vi "ImagerForFlowbit4.vi"() -> ()   [LabVIEW 2011]
uses:
  <vilib>/Platform/TimedLoop/XDataNode/timing_clust.ctl
  <vilib>/Platform/TimedLoop/XDataNode/nitl_modes.ctl
  <vilib>/Platform/TimedLoop/XDataNode/wakeup.ctl
  <vilib>/Analysis/1siggen.llb/Riffle Array (I32).vi
  <vilib>/Platform/TimedLoop/XDataNode/XDataNode.xnode
  <vilib>/Analysis/NI_AALBase.lvlib
  <vilib>/vision/NI_Vision_Development_Module.lvlib
  <vilib>/Platform/TimedLoop/XDataNode/XDNodeRunTimeDep.lvlib
panel:
  out "停止循环":bool
  in  "Stimuli":i64=5
  in  "选项卡控件":enum32{"前面板", "参数设置", "OnLineMap"}(tab)
  out "log":string
  out "Stim_ID":i32(listbox)=1
  in  "开始/暂停":bool=TRUE
  in  "停止":bool
  out "重排的 Stim ID":i32[](array[numeric]) caption="重排的{X}"
  out "block":i32
  out "队列中元素数量":i32
  out "Image 2":T1(plugin-control)
  in  "热图":bool
  out "循环持续时间":i64
  out "Recording":bool
  out "grabLoop":i32
  in  "address":i16=888 caption="地址" format="%.0x"
  in  "SaveParameter":bool
  in  "Pra_binType":enum16{"Extract", "Resample"}(ring)
  in  "Pra_FramesPerStim":i64=16
  in  "Pra_Blk目录":path=path "D:/Expt/test"
  in  "Pra_文件名":string="G4_E02"
  in  "Pra_TimeForPrepare(ms)":u32=1000
  in  "Pra_stim ID":u8[](array[numeric])=[0, 2, 4, 6, 8]
  in  "Pra_blk总数":i32=500
  in  "Pra_stim protocol":T2(array[ring])=[enum."prep stim", enum."wait respirator", enum."show stim", enum."recording data", enum."Blank stim", enum."ISI"]
  in  "Pra_blank stim":u8
  in  "Pra_wait（ms）":u32=10
  in  "Pra_ISI（ms）":u32=8000
  in  "Pra_FrameBin":i32=25
  in  "Pra_datatype":u16(ring)=13 items=["U8"=11, "I16"=12, "U32"=13, "SGL"=14]
  in  "FrameWidth":i64=704
  in  "FrameHeight":i64=576
  in  "LoadParameter":bool
  in  "Pra_bin":enum16{"1*1", "2*2"}(ring)
  in  "Pra_DR/R parameter":T3={"frame_zero_0"=0, "frame_zero_1"=1, "frame_0"=3, "frame_1"=15}
  in  "Pra_OnlineMap":cluster{"数组 1":i32[], "数组 2":i32[]}[](array[cluster])=[{"数组 1"=[2], "数组 2"=[6]}, {"数组 1"=[4], "数组 2"=[8]}, {"数组 1"=[2, 6], "数组 2"=[4, 8]}, {"数组 1"=[2, 4, 6, 8], "数组 2"=[0]}, {"数组 1"=[2, 4], "数组 2"=[6, 8]}]
  # "-"
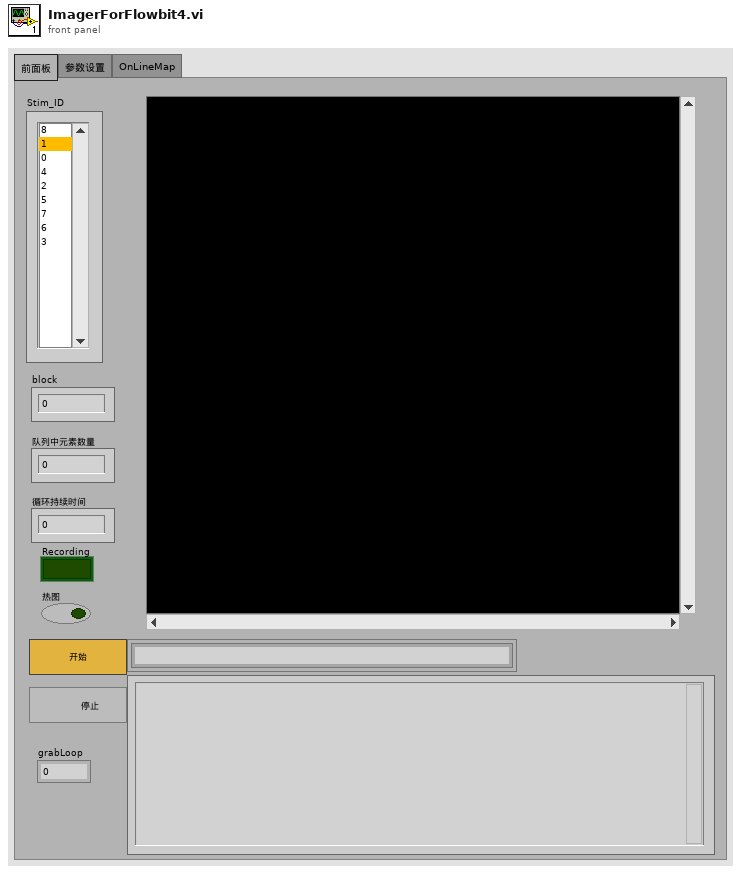
[diagram p1: front panel]
types:
  T1 = typedef "IMAQ Image.ctl" = refnum<image>
  T2 = enum16{"wait", "prep stim", "show stim", "wait respirator", "recording data", "Blank stim", "wait heart", "ISI", "DR/R", "wait calibrate", "openLightShutter", "closeLightShutter"}[]
  T3 = cluster{"frame_zero_0":i32, "frame_zero_1":i32, "frame_0":i32, "frame_1":i32}
  T4 = typedef "Image Type" = u32
  T5 = enum16{"Disable External Trigger", "Enable External Trigger"}
  T6 = enum32{"Auto Detect", "RoadRunner", "Raven", "R64"}
  T7 = typedef "XDNodeRunTimeDep.lvlib/timing_clust.ctl" = cluster{"Expected End [f-1]":u64, "Actual End [f-1]":u64, "Finished Late? [f-1]":bool, "Expected End [i-1]":u64, "Actual End [i-1]":u64, "Finished Late? [i-1]":bool, "Expected Start [i]":u64, "Actual Start [i]":u64, "Expected Start [f]":u64, "Actual Start [f]":u64, "Source Name":string, "Structure Name":string, "Period":i64, "Deadline":i64, "Offset":i64, "Start":i64, "Priority":i32, "Timeout":i32, "Mode":T8, "Wakeup Reason":T9, "Error":errorcluster, "Source Type":string, "Secondary Source Type":string, "Global End Time":u64, "Global Start Time":u64, "Frame Duration":u64, "Iteration Duration":u64, "Assigned CPU":i32, "I/O Scan Engine Mode":u32}
  T8 = typedef "XDNodeRunTimeDep.lvlib/nitl_modes.ctl" = enum32{"No Change", "Process missed periods, maintain original phase", "Discard missed periods, maintain original phase", "Process missed periods, ignore original phase", "Discard missed periods, ignore original phase"}
  T9 = typedef "XDNodeRunTimeDep.lvlib/wakeup.ctl" = enum32{"Normal", "Aborted", "Asynchronous wakeup", "Timing source error", "Timed loop error", "Timeout"}
  T10 = enum8{"Enabled", "Disabled", "Disabled and Grayed Out"}
  T11 = enum16{"open", "replace", "create", "open or create", "replace or create", "replace or create with confirmation"}
  T12 = enum16{"big-endian, network order", "native, host order", "little-endian"}
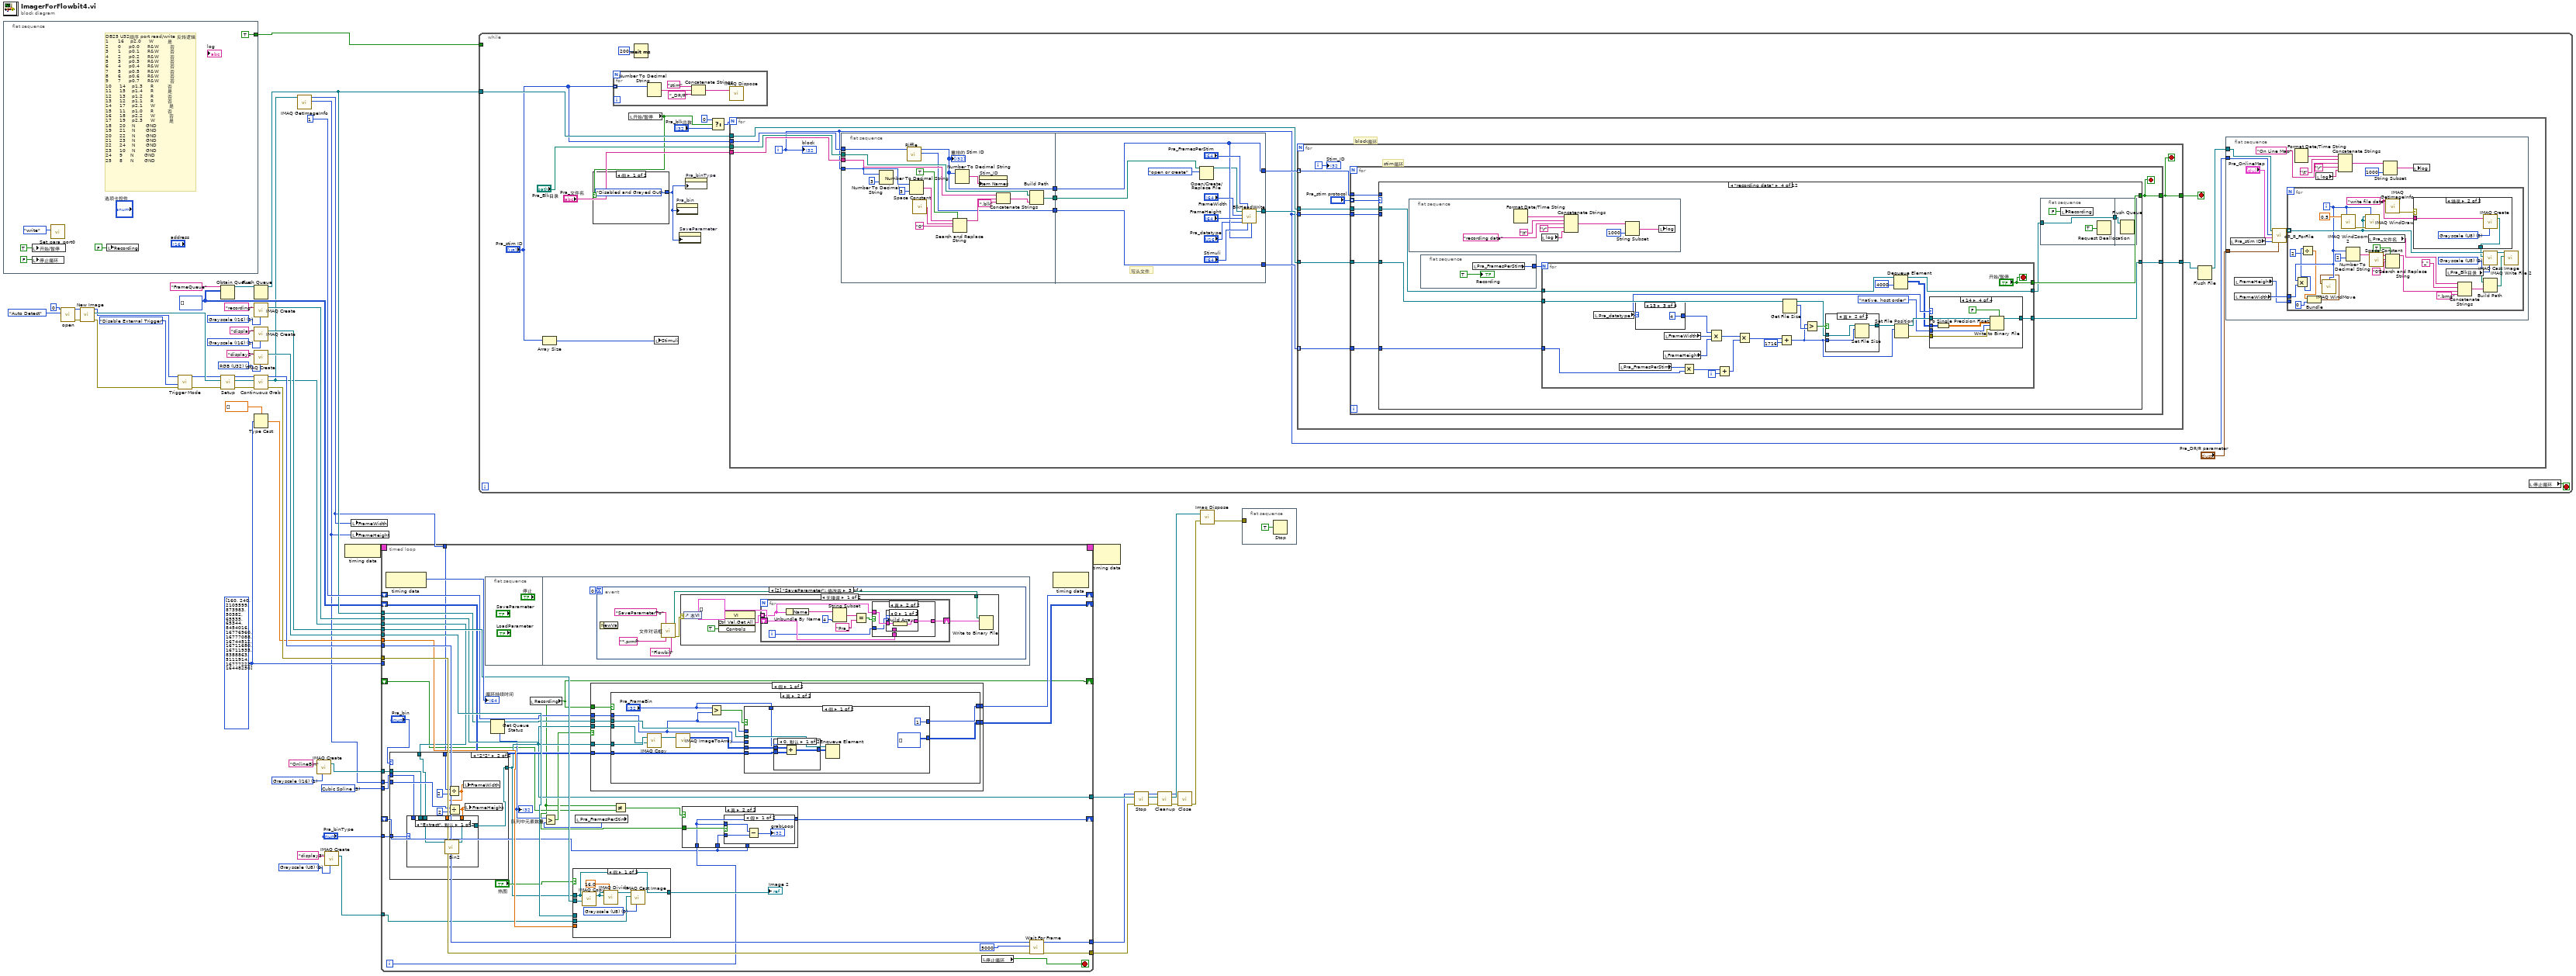
[diagram p0: block diagram]
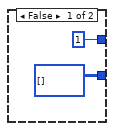
[diagram p4: hidden frame]
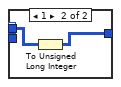
[diagram p5: hidden frame]
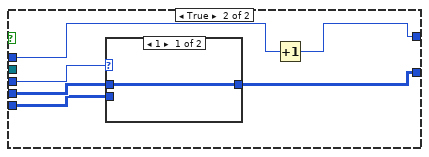
[diagram p6: hidden frame]
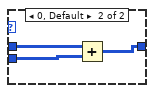
[diagram p7: hidden frame]
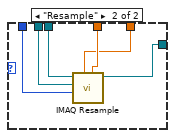
[diagram p10: hidden frame]
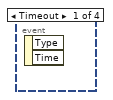
[diagram p11: hidden frame]
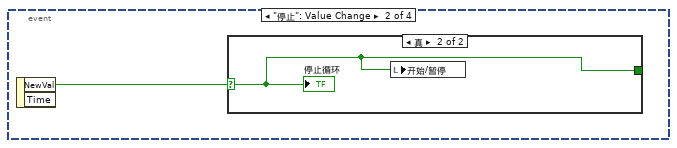
[diagram p12: hidden frame]
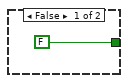
[diagram p13: hidden frame]
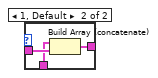
[diagram p15: hidden frame]
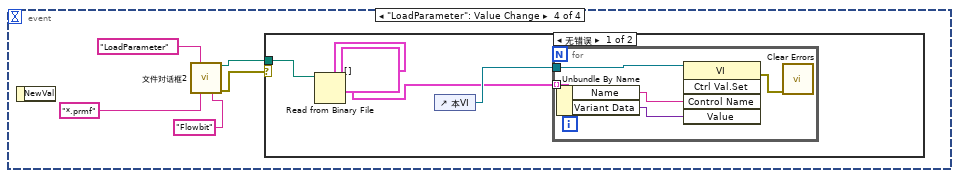
[diagram p17: hidden frame]
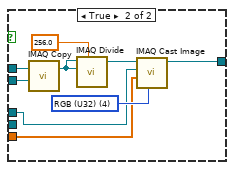
[diagram p19: hidden frame]
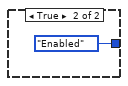
[diagram p20: hidden frame]
diagram:
  w3 = T4 0 items=["Grayscale (U8)", "Grayscale (I16)", "Grayscale (SGL)", "Complex (CSG)", "RGB (U32)", "HSL (U32)", "RGB (U64)", "Grayscale (U16)"] ("Image Type")
  w8 = u32 3 items=["Zero Order", "Bi-Linear", "Quadratic", "Cubic Spline"] ("Interpolation Type")
  w10 = T4 1 items=["Grayscale (U8)", "Grayscale (I16)", "Grayscale (SGL)", "Complex (CSG)", "RGB (U32)", "HSL (U32)", "RGB (U64)", "Grayscale (U16)"] ("Image Type")
  w13 = u32[][] []
  w23 = T4 4 items=["Grayscale (U8)", "Grayscale (I16)", "Grayscale (SGL)", "Complex (CSG)", "RGB (U32)", "HSL (U32)", "RGB (U64)", "Grayscale (U16)"] ("Image Type")
  w21 = u32[] [160, 240, 2105599, 873983, 50382, 65535, 65344, 8454016, 16776960, 16777088, 16744512, 16711680, 16711935, 8388863, 5111914, 16777222, 16448250] ("数组")
  w27 = T4 1 items=["Grayscale (U8)", "Grayscale (I16)", "Grayscale (SGL)", "Complex (CSG)", "RGB (U32)", "HSL (U32)", "RGB (U64)", "Grayscale (U16)"] ("Image Type")
  w28 = T4 1 items=["Grayscale (U8)", "Grayscale (I16)", "Grayscale (SGL)", "Complex (CSG)", "RGB (U32)", "HSL (U32)", "RGB (U64)", "Grayscale (U16)"] ("Image Type")
  n1 = flat-sequence {
    tunnel: [TRUE ("Zoom to Fit Mode")] -> w16
    frame #0 {
      # "DB25\tU32顺序\tport\tread/write\t反转逻辑\n1\t     16\t   p2.0    \tW\t        是\n2\t     0    \tp0.0\t   \tR&W\t      否\n3\t     1\t\t   p0.1\t   \tR&W      \t否\n4\t\t    2\t   \tp0.2   \t\tR&W      \t否\n5\t\t    3\t\t   p0.3   \t\tR&W\t      否\n6\t\t    4\t   \tp0.4   \t\tR&W      \t否\n7\t\t    5\t   \tp0.5   \t\tR&W      \t否\n8\t\t    6\t   \tp0.6\t   \tR&W      \t否\n9\t    \t7\t   \tp0.7\t   \tR&W\t      否\n10\t    14   \tp1.3   \t\tR        \t否\n11\t   \t15   \tp1.4   \t\tR        \t是\n12\t   \t13   \tp1.2\t   \tR        \t否\n13    \t12   \tp1.1\t   \tR        \t否\n14     17   \tp2.1\t   \tW        \t是\n15    \t11   \tp1.0   \t\tR\t        否\n16    \t18   \tp2.2   \t\tW        \t否\n17    \t19\t   p2.3   \t\tW\t        是\n18    \t20   \tN   \t  \tGND\t\n19    \t21   \tN   \t  \tGND\t\n20\t    22\t   N\t  \t  \tGND\t\n21\t    23\t   N  \t  \t\tGND\t\n22\t    24\t   N  \t  \t\tGND\t\n23    \t10   \tN  \t  \t\tGND\t\n24    \t9\t    N  \t  \t\tGND\t\n25\t    8    \tN  \t  \t\tGND"
      n2 = local write "开始/暂停"(TRUE ("开始/暂停")) -> ()
      n3 = local write "停止循环"(FALSE ("开始/暂停")) -> ()
      n4 = call "Set_para_port0.vi"("R or W"=enum16{"read", "write"}."write") -> ()  [unwired: 9 in, 2 out]
      n5 = local write "Recording"(FALSE ("Recording")) -> ()
    }
  }
  n6 = call <vilib>:"open.vi"("Board Type"=T6."Auto Detect", "Board Number"=u32 0) -> ("error out"=w44:errorcluster, "RefBrdOut"=w39:u32)  [unwired: 2 in, 5 out]
  n7 = call <vilib>:"New Image.vi"("RefBrdIn"=w39, "error in"=w44) -> ("RefBrdOut"=w38:u32, "Image"=w53:T1, "error out"=w45:errorcluster)  [unwired: 6 in]
  n8 = call <vilib>:"Trigger Mode.vi"("RefBrdIn"=w38, "Trigger Mode"=T5."Disable External Trigger", "error in (no error)"=w45) -> ("RefBrdOut"=w37:u32, "error out"=w46:errorcluster)  [unwired: 6 in]
  n9 = Obtain Queue(name (unnamed)="FrameQueue" ("名称（未命名）"), element data type=w13) -> (queue out=w17:refnum<queue>)  [unwired: 3 in, 2 out]
  n10 = call <vilib>:"Setup.vi"("error in"=w46, "Image In"=w53, "RefBrdIn"=w37) -> ("error out"=w41:errorcluster, "Image"=w42:T1, "RefBrdOut"=w36:u32)  [unwired: 6 in]
  n11 = Flush Queue(queue=w17) -> (queue out=w14:refnum<queue>)  [unwired: 1 in, 2 out]
  n12 = call "IMAQ Create"("Image Name"="recording", "Image Type"=w28) -> ("New Image"=w30:T1)  [unwired: 3 in, 1 out]
  n13 = call "IMAQ Create"("Image Name"="display", "Image Type"=w27) -> ("New Image"=w25:T1)  [unwired: 3 in, 1 out]
  n14 = call "IMAQ Create"("Image Name"="display2", "Image Type"=w23) -> ("New Image"=w22:T1)  [unwired: 3 in, 1 out]
  n15 = call <vilib>:"Continuous Grab.vi"("error in (no error)"=w41, "Image In"=w42, "RefBrdIn"=w36) -> ("error out"=w40:errorcluster, "Image"=w4:T1, "RefBrdOut"=w35:u32)  [unwired: 6 in]
  n16 = Type Cast(type=sgl[] [] ("单精度浮点"), x=w21) -> (*(type *) &x=w19:sgl[])
  n17 = call "IMAQ GetImageInfo"("Image"=w4) -> ("Y Resolution"=w6:i32, "X Resolution"=w7:i32)  [unwired: 3 in, 6 out]
  n18 = call "IMAQ Create"("Image Name"="OnlineBin", "Image Type"=w10) -> ("New Image"=w9:T1)  [unwired: 3 in, 1 out]
  n19 = call "IMAQ Create"("Image Name"="display3", "Image Type"=w3) -> ("New Image"=w1:T1)  [unwired: 3 in, 1 out]
  n20 = node-c288() -> (w57:T7)
  n21 = local write "FrameWidth"(w7) -> ()
  n22 = local write "FrameHeight"(w6) -> ()
  n23 = timed-loop {
    tunnel: [w77] -> w52
    tunnel: [w99] -> w47
    tunnel: w4 -> [w78]
    tunnel: w40 -> [w98]
    tunnel: w35 -> [w97]
    tunnel: [w96] -> w34
    timing: w57 -> [_]
    timing-out: [_] -> w56
    tunnel: w30 -> [w87]
    tunnel: w14 -> [w82]
    tunnel: w25 -> [w92]
    tunnel: w21 -> [_]
    tunnel: w22 -> [w91]
    tunnel: w19 -> [w90]
    shift-right: [w85] -> _
    shift-left: 1 -> [w86]
    shift-right: [w84] -> _
    shift-left: w13 -> [w83]
    tunnel: w9 -> [w80]
    tunnel: w8 -> [w79]
    tunnel: w7 -> [w75]
    tunnel: w6 -> [w74]
    tunnel: "Pra_binType" -> [w73]
    shift-right: [w65] -> _
    shift-left: _ -> [w69]
    shift-right: [w66] -> _
    shift-left: _ -> [w64]
    tunnel: w1 -> [w63]
    i -> [w67]
    stop <- w93 stop-if-true
    n24 = node-c288() -> (→"循环持续时间":i64)  [unwired: 1 in]
    n25 = case shown="\"2*2\"" "Pra_bin" {
      tunnel: w80 -> [_ w159]
      tunnel: w79 -> [_ w154]
      tunnel: w78 -> [w152 w158]
      tunnel: [w152 w157] -> w77
      tunnel: w75 -> [_ w163]
      tunnel: w74 -> [_ w160]
      tunnel: w73 -> [_ w153]
      frame "1*1", Default {
      }
      frame "2*2" {
        n26 = Divide(x=w163, y=2) -> (x/y=w156:dbl)
        n27 = Divide(x=w160, y=2) -> (x/y=w155:dbl)
        n28 = case shown="\"Extract\", 默认" w153 {
          tunnel: w159 -> [_ w170]
          tunnel: w158 -> [w165 w171]
          tunnel: [w164 w167] -> w157
          tunnel: w156 -> [_ w169]
          tunnel: w155 -> [_ w168]
          tunnel: w154 -> [_ w166]
          frame "Extract", Default {
            n29 = call "Bin2.vi"("Image Src"=w165) -> ("Image"=w164:T1)  [unwired: 10 in]
          }
          frame "Resample" {
            n30 = call "IMAQ Resample"("X Resolution"=w169, "Y Resolution"=w168, "Interpolation Type"=w166, "Image Dst"=w170, "Image Src"=w171) -> ("Image Dst Out"=w167:T1)  [unwired: 5 in, 1 out]
          }
        }
        n31 = local write "FrameWidth"(w156) -> ()
        n32 = local write "FrameHeight"(w155) -> ()
      }
    }
    n33 = flat-sequence {
      frame #0 {
      }
      frame #1 {
        n34 = event shown="[2] \"SaveParameter\": 值改变" {
          selector: _ -> [_ _ _ _]
          dyn-events: _ -> [_ _ _ _]
          timeout: 0 -> [_ _ _ _]
          event Timeout {
            n35 = event-data() -> ()  [unwired: 1 in, 2 out]
          }
          event "停止": Value Change {
            n36 = event-data() -> ("NewVal"=w173:bool)  [unwired: 1 in, 1 out]
            n37 = case shown="真" w173 {
              selector: w173 -> [_ w175]
              tunnel: [FALSE w175] -> _
              frame False {
              }
              frame True {
                n38 = local write "开始/暂停"(w175) -> ()
                "停止循环" <- w175
              }
            }
          }
          event "SaveParameter": Value Change {
            n39 = event-data() -> ()  [unwired: 1 in, 1 out]
            n40 = call "文件对话框"("prompt"="SaveParameterTo", "pattern (all files)"="*.prmf", "pattern label"="Flowbit") -> ("selected path"=w177:path, "error out"=w179:errorcluster)  [unwired: 9 in, 2 out]
            n41 = case shown="无错误" w179 {
              tunnel: w177 -> [w182 _]
              frame No Error {
                n42 = control-ref of="本VI"() -> (w186:refnum<vi>)
                n43 = invoke class="VI" method="Ctrl Val.Get All"(reference=w186, "Controls"=TRUE ("输入控件")) -> ("Get All Control Values Variant"=w185:cluster{"Name":string, "Variant Data":variant}[])  [unwired: 2 in, 3 out]
                n44 = for {
                  tunnel: w185 -> [w190] mode=indexing
                  shift-right: [w189] -> w183
                  shift-left: cluster{"Name":string, "Variant Data":variant}[] [] -> [w188]
                  i -> [w187]
                  n45 = Unbundle By Name(w190) -> ("Name"=w195:string)
                  n46 = String Subset(string=w195, length (rest)=4 ("长度（剩余）")) -> (substring=w193:string)  [unwired: 1 in]
                  n47 = Equal?(x=w193, y="Pra_") -> (x = y?=w191:bool)
                  n48 = case shown="真" w191 {
                    tunnel: w190 -> [_ w200]
                    tunnel: [w196 w199] -> w189
                    tunnel: w188 -> [w196 w198]
                    tunnel: w187 -> [_ w197]
                    frame False {
                    }
                    frame True {
                      n49 = case shown="0" w197 {
                        tunnel: w200 -> [w202 w205]
                        tunnel: [w201 w204] -> w199
                        tunnel: w198 -> [_ w203]
                        frame 0 {
                          n50 = Build Array(w202) -> (w201:cluster{"Name":string, "Variant Data":variant}[])
                        }
                        frame 1, Default {
                          n51 = Build Array (concatenate)(w203, w205) -> (w204:cluster{"Name":string, "Variant Data":variant}[])
                        }
                      }
                    }
                  }
                }
                n52 = Write to Binary File(file (use dialog)=w182, data=w183) -> ()  [unwired: 4 in, 3 out]
              }
              frame Error {
              }
            }
          }
          event "LoadParameter": Value Change {
            n53 = event-data() -> ()  [unwired: 1 in, 1 out]
            n54 = call "文件对话框2"("prompt"="LoadParameter", "pattern (all files)"="*.prmf", "pattern label"="Flowbit") -> ("selected path"=w206:path, "error out"=w207:errorcluster)  [unwired: 9 in, 2 out]
            n55 = case shown="无错误" w207 {
              tunnel: w206 -> [w214 _]
              frame No Error {
                n56 = Read from Binary File(5:cluster{"Name":string, "Variant Data":variant}[] [], 11:w214) -> (2:w211:cluster{"Name":string, "Variant Data":variant}[])  [unwired: 4 in, 3 out]
                n57 = control-ref of="本VI"() -> (w212:refnum<vi>)
                n58 = for {
                  tunnel: w212 -> [w219]
                  tunnel: w211 -> [w218] mode=indexing
                  n59 = Unbundle By Name(w218) -> ("Name"=w217:string, "Variant Data"=w216:variant)
                  n60 = invoke class="VI" method="Ctrl Val.Set"(reference=w219, "Control Name"=w217, "Value"=w216) -> (error out=w215:errorcluster)  [unwired: 2 in, 4 out]
                  n61 = call <vilib>:"Clear Errors.vi"("error in (no error)"=w215) -> ()  [unwired: 6 in, 1 out]
                }
              }
              frame Error {
              }
            }
          }
        }
      }
    }
    n62 = Get Queue Status(queue=w82) -> (queue out=w81:refnum<queue>, # elements in queue=w72:i32)  [unwired: 2 in, 6 out]
    "队列中元素数量" <- w72
    n63 = local read "Recording"() -> (w65:bool)
    n64 = case shown="假" "热图" {
      tunnel: w92 -> [w226 w234]
      tunnel: w77 -> [w220 w232]
      tunnel: [w220 w231] -> w89
      tunnel: w91 -> [_ w229]
      tunnel: w90 -> [_ w228]
      tunnel: w63 -> [w224 _]
      frame False {
        w225 = T4 0 items=["Grayscale (U8)", "Grayscale (I16)", "Grayscale (SGL)", "Complex (CSG)", "RGB (U32)", "HSL (U32)", "RGB (U64)", "Grayscale (U16)"] ("Image Type")
        n65 = call "IMAQ Copy"("Image Dst"=w226, "Image Src"=w220) -> ("Image Dst Out"=w223:T1)  [unwired: 4 in, 1 out]
        n66 = call "IMAQ Divide"("Image Src A"=w223, "Constant"=sgl 16.0, "Image Dst"=w223) -> ("Image Dst Out"=w221:T1)  [unwired: 4 in, 1 out]
        n67 = call "IMAQ Cast Image"("Image Type"=w225, "Image Dst"=w224, "Image Src"=w221) -> ()  [unwired: 7 in, 2 out]
      }
      frame True {
        w230 = T4 4 items=["Grayscale (U8)", "Grayscale (I16)", "Grayscale (SGL)", "Complex (CSG)", "RGB (U32)", "HSL (U32)", "RGB (U64)", "Grayscale (U16)"] ("Image Type")
        n68 = call "IMAQ Copy"("Image Dst"=w234, "Image Src"=w232) -> ("Image Dst Out"=w233:T1)  [unwired: 4 in, 1 out]
        n69 = call "IMAQ Divide"("Image Src A"=w233, "Constant"=sgl 256.0, "Image Dst"=w233) -> ("Image Dst Out"=w227:T1)  [unwired: 4 in, 1 out]
        n70 = call "IMAQ Cast Image"("Image Type"=w230, "Lookup Table"=w228, "Image Dst"=w229, "Image Src"=w227) -> ("Image Dst Out"=w231:T1)  [unwired: 6 in, 1 out]
      }
    }
    "Image 2" <- w89
    n71 = local read "Pra_FramesPerStim"() -> (w71:i64)
    n72 = Greater?(x=w72, y=w71) -> (0:w70:bool)
    n73 = case shown="假" w70 {
      tunnel: w65 -> [w114 _]
      tunnel: w87 -> [w113 _]
      tunnel: w86 -> [w112 w150]
      tunnel: [w111 w150] -> w85
      tunnel: [w110 w151] -> w84
      tunnel: w83 -> [w109 w151]
      tunnel: w81 -> [w108 _]
      tunnel: w77 -> [w107 _]
      frame False {
        n74 = case shown="真" w114 {
          tunnel: w108 -> [_ w122]
          tunnel: w107 -> [_ w127]
          tunnel: w113 -> [_ w126]
          tunnel: w112 -> [_ w118]
          tunnel: [1 w123] -> w111
          tunnel: w109 -> [_ w119]
          tunnel: [u32[][] [] w121] -> w110
          frame False {
          }
          frame True {
            n75 = call "IMAQ Copy"("Image Dst"=w126, "Image Src"=w127) -> ("Image Dst Out"=w125:T1)  [unwired: 4 in, 1 out]
            n76 = call "IMAQ ImageToArray"("Image"=w125) -> ("Image Pixels (I16)"=w120:i16[][])  [unwired: 3 in, 4 out]
            n77 = Greater?(x="Pra_FrameBin", y=w118) -> (0:w124:bool)
            n78 = case shown="假" w124 {
              tunnel: w118 -> [_ w141]
              tunnel: [1 w140] -> w123
              tunnel: w122 -> [w133 _]
              tunnel: [u32[][] [] w143] -> w121
              tunnel: w120 -> [w132 w145]
              tunnel: w119 -> [w131 w144]
              tunnel: w118 -> [_ w142]
              tunnel: "Pra_FrameBin" -> [w128 _]
              frame False {
                n79 = case shown="0, 默认" w128 {
                  tunnel: w132 -> [w137 w139]
                  tunnel: w131 -> [w136 _]
                  tunnel: [w135 w138] -> w129
                  frame 0, Default {
                    n80 = Add(x=w137, y=w136) -> (x+y=w135:u32[][])
                  }
                  frame 1 {
                    n81 = To Unsigned Long Integer(number=w139) -> (unsigned 32bit integer=w138:u32[][])
                  }
                }
                n82 = Enqueue Element(queue=w133, element=w129) -> ()  [unwired: 2 in, 3 out]
              }
              frame True {
                n83 = case shown="1" w142 {
                  tunnel: w145 -> [w146 w149]
                  tunnel: w144 -> [_ w148]
                  tunnel: [w146 w147] -> w143
                  frame 1 {
                  }
                  frame 0, Default {
                    n84 = Add(x=w149, y=w148) -> (x+y=w147:u32[][])
                  }
                }
                n85 = Increment(x=w141) -> (x+1=w140:i32)
              }
            }
          }
        }
      }
      frame True {
      }
    }
    n86 = Not Equal?(x=w65, y=w69) -> (x != y?=w68:bool)
    n87 = case shown="真" w68 {
      tunnel: w67 -> [_ w101]
      tunnel: [w100 w101] -> w66
      tunnel: w64 -> [w100 w102]
      tunnel: w65 -> [_ w103]
      tunnel: w64 -> [_ _]
      frame False {
      }
      frame True {
        n88 = case shown="假" w103 {
          tunnel: w102 -> [w105 _]
          tunnel: w101 -> [w104 _]
          frame False {
            n89 = Subtract(x=w104, y=w105) -> (x-y=→"grabLoop":i32)
          }
          frame True {
          }
        }
      }
    }
    n90 = local read "停止循环"() -> (w93:bool)
    n91 = call <vilib>:"Wait For Frame.vi"("error in (no error)"=w98, "Timeout (mS)"=u32 5000, "RefBrdIn"=w97) -> ("error out"=w99:errorcluster, "RefBrdOut"=w96:u32)  [unwired: 7 in]
    n92 = node-c288() -> ()  [unwired: 1 in, 1 out]
  }
  n93 = while {
    tunnel: w16 -> [_]
    tunnel: w14 -> [w245]
    stop <- w249 stop-if-true
    n94 = Array Size(array="Pra_stim ID") -> (size(s)=w242:i32)
    n95 = for {
      tunnel: "Pra_stim ID" -> [w254] mode=indexing
      n96 = Number To Decimal String(number=w254) -> (decimal integer string=w255:string)  [unwired: 1 in]
      n97 = Concatenate Strings("stim" ("字符串"), w255, "_DR/R" ("字符串")) -> (w253:string)
      n98 = call "IMAQ Dispose"("Image"=w253) -> ()  [unwired: 5 in, 1 out]
    }
    n99 = local read "开始/暂停"() -> (w240:bool)
    n100 = case shown="假" w240 {
      tunnel: [T10."Disabled and Grayed Out" ("禁用") T10."Enabled" ("禁用")] -> w239
      frame False {
      }
      frame True {
      }
    }
    n101 = Wait (ms)(milliseconds to wait=u32 200 ("等待时间（毫秒）")) -> ()  [unwired: 1 out]
    n102 = local write "Stimuli"(w242) -> ()
    n103 = property on="Pra_bin" class="Enum (严格)"("DisabledEnum"=w239) -> ()  [unwired: 2 in, 2 out]
    n104 = property on="SaveParameter" class="Bool"("DisabledEnum"=w239) -> ()  [unwired: 2 in, 2 out]
    n105 = property on="Pra_binType" class="Enum (严格)"("DisabledEnum"=w239) -> ()  [unwired: 2 in, 2 out]
    n106 = Select(t=0, s=w240, f="Pra_blk总数") -> (s? t:f=w246:i32)
    n107 = for {
      N: w246 -> [_]
      tunnel: "Pra_stim ID" -> [w267]
      tunnel: "Pra_文件名" -> [w272]
      tunnel: "Pra_Blk目录" -> [w271]
      tunnel: w245 -> [w265]
      i -> [w263]
      stop <- w268 stop-if-true
      # "block循环"
      n108 = flat-sequence {
        tunnel: [w325] -> w262
        tunnel: w263 -> [w324]
        tunnel: w272 -> [w330]
        tunnel: w271 -> [w326]
        tunnel: w267 -> [w320]
        tunnel: [w322] -> w261
        tunnel: [w321] -> w260
        tunnel: w262 -> [w341]
        tunnel: [w343] -> w270
        tunnel: w261 -> [w342]
        tunnel: [w342] -> w269
        tunnel: w260 -> [w337]
        tunnel: [w337] -> w266
        frame #0 {
          n109 = Number To Decimal String(number=w324, width (-)=i16 3 ("宽度(-)")) -> ()  [unwired: 1 out]
          n110 = call-poly <vilib>:"Riffle.vi"("X"=w320) -> ("Riffled Index"=w321:i32[], "Riffled {X}"=w322:i32[])  [unwired: 8 in, 1 out]
          "重排的 Stim ID" <- w322
          n111 = Number To Decimal String(number=w324, width (-)=i16 3 ("宽度(-)")) -> (decimal integer string=w332:string)
          n112 = call <vilib>:"Space Constant.vi"() -> ("String"=w333:string)
          n113 = Search and Replace String(replace all?=TRUE ("替换全部？(F)"), input string=w332, search string=w333, replace string="0" ("替换字符串(\"\")")) -> (result string=w329:string)  [unwired: 4 in, 3 out]
          n114 = Number To Decimal String(number=w322) -> (decimal integer string=w323:string[])  [unwired: 1 in]
          n115 = property on="Stim_ID" class="LstBox (严格)"("Item Names"=w323) -> ()  [unwired: 2 in, 2 out]
          n116 = Concatenate Strings(w330, w329, ".blk" ("字符串")) -> (w327:string)
          n117 = Build Path(base path=w326, name or relative path=w327) -> (appended path=w325:path)
        }
        frame #1 {
          # "写头文件"
          n118 = Open/Create/Replace File(file path (use dialog)=w341, operation (0:open)=T11."open or create" ("操作(0:open)")) -> (refnum out=w339:refnum<file>)  [unwired: 4 in, 2 out]
          n119 = call "BlkHeadWrite.vi"("SequenceOfID"=w342, "Stimuli"="Stimuli", "FramesPerStim"="Pra_FramesPerStim", "datatype"="Pra_datatype", "FrameHeight"="FrameHeight", "FrameWidth"="FrameWidth", "引用句柄输入"=w339) -> ("引用句柄输出"=w343:refnum<file>)  [unwired: 4 in]
        }
      }
      n120 = for {
        tunnel: w270 -> [w356]
        tunnel: [w354] -> w259
        tunnel: w266 -> [w355] mode=indexing
        tunnel: w269 -> [w353] mode=indexing
        tunnel: [w352] -> w268
        tunnel: w263 -> [w349]
        tunnel: w265 -> [w348]
        i -> [w351]
        stop <- w352 stop-if-true
        # "stim循环"
        n121 = for {
          tunnel: w355 -> [w363]
          tunnel: w353 -> [w361]
          tunnel: [w359] -> w352
          tunnel: "Pra_stim protocol" -> [w360] mode=indexing
          tunnel: w356 -> [w364]
          tunnel: [w362] -> w354
          tunnel: w349 -> [w358]
          tunnel: w348 -> [w357]
          stop <- w359 stop-if-true
          n122 = case shown="\"recording data\"" w360 {
            tunnel: w364 -> [w367 w385 w399 w416 w494 w507 w521 w536 w558 w568 w570 w582]
            tunnel: w363 -> [_ _ _ w415 _ _ _ w534 _ _ _ _]
            tunnel: [w367 w385 w399 w414 w494 w507 w521 w536 w558 w568 w570 w582] -> w362
            tunnel: w361 -> [w365 _ _ _ _ _ _ _ _ _ _ _]
            tunnel: [w368 w386 w400 w417 w495 w508 w522 w535 w559 w569 w571 w583] -> w359
            tunnel: w358 -> [_ _ _ _ _ _ _ w533 _ _ _ _]
            tunnel: w357 -> [_ _ _ w412 _ _ _ _ _ _ _ _]
            frame "prep stim" {
              n123 = Number To Boolean Array(number=w365) -> (Boolean array=w369:bool[])
              n124 = flat-sequence {
                tunnel: w369 -> [w380]
                tunnel: [w380] -> w366
                tunnel: w365 -> [w379]
                tunnel: w366 -> [w383]
                frame #0 {
                  n125 = Number To Decimal String(number=w379) -> (decimal integer string=w376:string)  [unwired: 1 in]
                  n126 = Format Date/Time String() -> (date/time string=w378:string)  [unwired: 3 in]
                  n127 = local read "log"() -> (w372:string)
                  n128 = Concatenate Strings(w378, "\t", "prep stim ID=" ("字符串"), w376, "\r", w372) -> (w374:string)
                  n129 = String Subset(string=w374, length (rest)=1000 ("y")) -> (substring=w373:string)  [unwired: 1 in]
                  n130 = local write "log"(w373) -> ()
                }
                frame #1 {
                  n131 = call "Write_para_port0.vi"("port0（8元素）"=w383) -> ()  [unwired: 10 in, 1 out]
                  n132 = call "Write_para_port2_singalChange.vi"("索引"=0, "布尔"=TRUE) -> ()  [unwired: 9 in, 1 out]
                }
                frame #2 {
                  n133 = Wait (ms)(milliseconds to wait="Pra_TimeForPrepare(ms)") -> ()  [unwired: 1 out]
                }
              }
              n134 = local read "开始/暂停"() -> (w368:bool)
            }
            frame "wait respirator" {
              n135 = while {
                stop <- w396 stop-if-true
                # "this step will return true if pallel port doesn't connect any signal.That means this loop only run once."
                n136 = call "read_para_port1.vi"() -> ("port1（5元素）"=w398:bool[])  [unwired: 10 in, 1 out]
                n137 = Index Array(array=w398, index=3 ("索引")) -> (element=w396:bool)
                n138 = Wait (ms)(milliseconds to wait=u32 5 ("等待时间（毫秒）")) -> ()  [unwired: 1 out]
              }
              n139 = flat-sequence {
                frame #0 {
                  n140 = Format Date/Time String() -> (date/time string=w394:string)  [unwired: 3 in]
                  n141 = local read "log"() -> (w389:string)
                  n142 = Concatenate Strings(w394, "\t", "wait respiratory" ("字符串"), "\r", w389) -> (w391:string)
                  n143 = String Subset(string=w391, length (rest)=1000 ("y")) -> (substring=w390:string)  [unwired: 1 in]
                  n144 = local write "log"(w390) -> ()
                }
              }
              n145 = local read "开始/暂停"() -> (w386:bool)
            }
            frame "show stim" {
              n146 = flat-sequence {
                frame #0 {
                  n147 = call "Write_para_port2_singalChange.vi"("索引"=0, "布尔"=FALSE) -> ()  [unwired: 9 in, 1 out]
                }
              }
              n148 = flat-sequence {
                frame #0 {
                  n149 = Format Date/Time String() -> (date/time string=w408:string)  [unwired: 3 in]
                  n150 = local read "log"() -> (w403:string)
                  n151 = Concatenate Strings(w408, "\t", "show stim" ("字符串"), "\r", w403) -> (w405:string)
                  n152 = String Subset(string=w405, length (rest)=1000 ("y")) -> (substring=w404:string)  [unwired: 1 in]
                  n153 = local write "log"(w404) -> ()
                }
              }
              n154 = local read "开始/暂停"() -> (w400:bool)
            }
            frame "recording data" {
              n155 = flat-sequence {
                frame #0 {
                  n156 = Format Date/Time String() -> (date/time string=w432:string)  [unwired: 3 in]
                  n157 = local read "log"() -> (w427:string)
                  n158 = Concatenate Strings(w432, "\t", "recording data" ("字符串"), "\r", w427) -> (w429:string)
                  n159 = String Subset(string=w429, length (rest)=1000 ("y")) -> (substring=w428:string)  [unwired: 1 in]
                  n160 = local write "log"(w428) -> ()
                }
              }
              n161 = flat-sequence {
                tunnel: [w420] -> w418
                frame #0 {
                  n162 = local read "Pra_FramesPerStim"() -> (w420:i64)
                  "Recording" <- TRUE ("Recording")
                }
              }
              n163 = for {
                N: w418 -> [_]
                tunnel: ["开始/暂停"] -> w417
                tunnel: w416 -> [w458]
                tunnel: w415 -> [w442]
                tunnel: [w450] -> w414
                tunnel: [w449] -> w413
                tunnel: w412 -> [w434]
                i -> [w440]
                stop <- "开始/暂停" stop-if-true
                n164 = local read "Pra_datatype"() -> (w454:u16)
                n165 = local read "Pra_FramesPerStim"() -> (w443:i64)
                n166 = case shown="13" w454 {
                  tunnel: [i64 1 i64 2 i64 4 i64 4] -> w446
                  frame 11, Default {
                  }
                  frame 12 {
                  }
                  frame 13 {
                  }
                  frame 14 {
                  }
                }
                n167 = local read "FrameHeight"() -> (w444:i64)
                n168 = local read "FrameWidth"() -> (w445:i64)
                n169 = Multiply(x=w443, y=w442) -> (x*y=w441:i64)
                n170 = Compound Arithmetic op=MULTIPLY(w446, w445, w444) -> (w438:i64)
                n171 = Add(x=w441, y=w440) -> (x+y=w439:i64)
                n172 = Multiply(x=w438, y=w439) -> (x*y=w437:i64)
                n173 = Add(x=w437, y=i64 1716 ("x")) -> (x+y=w435:i64)
                n174 = Get File Size(file=w458) -> (refnum out=w451:refnum<file>, size (in bytes)=w447:i64)  [unwired: 1 in, 1 out]
                n175 = Greater?(x=w435, y=w447) -> (0:w452:bool)
                n176 = case shown="真" w452 {
                  tunnel: w435 -> [_ w489]
                  tunnel: w451 -> [w486 w488]
                  tunnel: [w486 w487] -> w453
                  frame False {
                  }
                  frame True {
                    n177 = Set File Size(6:w489, 7:w488) -> (3:w487:refnum<file>)  [unwired: 1 in, 1 out]
                  }
                }
                n178 = Dequeue Element(queue=w434, timeout in ms (-1)=4000 ("超时毫秒(-1)")) -> (queue out=w449:refnum<queue>, element=w433:u32[][])  [unwired: 1 in, 2 out]
                n179 = Set File Position(offset (in bytes) (0)=w435, refnum=w453) -> (refnum out=w457:refnum<file>, error out=w455:errorcluster)  [unwired: 2 in]
                n180 = case shown="14" w454 {
                  tunnel: w433 -> [w461 w468 w473 w479]
                  tunnel: w457 -> [w465 w469 w476 w481]
                  tunnel: T12."native, host order" ("字节顺序(0:big-endian, network order)") -> [w464 w470 w474 w482]
                  tunnel: w455 -> [w463 _ w475 w483]
                  tunnel: [w462 w471 w477 w484] -> w450
                  frame 11, Default {
                    n181 = To Unsigned Byte Integer(number=w461) -> (unsigned 8bit integer=w460:u8[][])
                    n182 = Write to Binary File(file (use dialog)=w465, data=w460, error in=w463, 5:FALSE ("预置数组或字符串大小？(T)"), 9:w464) -> (refnum out=w462:refnum<file>)  [unwired: 1 in, 2 out]
                  }
                  frame 12 {
                    n183 = To Unsigned Word Integer(number=w468) -> (unsigned 16bit integer=w467:u16[][])
                    n184 = Write to Binary File(file (use dialog)=w469, data=w467, 5:FALSE ("预置数组或字符串大小？(T)"), 9:w470) -> (refnum out=w471:refnum<file>)  [unwired: 2 in, 2 out]
                  }
                  frame 13 {
                    n185 = Write to Binary File(file (use dialog)=w476, data=w473, error in=w475, 5:FALSE ("预置数组或字符串大小？(T)"), 9:w474) -> (refnum out=w477:refnum<file>)  [unwired: 1 in, 2 out]
                  }
                  frame 14 {
                    n186 = To Single Precision Float(number=w479) -> (single precision float=w480:sgl[][])
                    n187 = Write to Binary File(file (use dialog)=w481, data=w480, error in=w483, 5:FALSE ("预置数组或字符串大小？(T)"), 9:w482) -> (refnum out=w484:refnum<file>)  [unwired: 1 in, 2 out]
                  }
                }
              }
              n188 = flat-sequence {
                tunnel: w413 -> [w421]
                tunnel: [w421] -> w411
                tunnel: w411 -> [w424]
                frame #0 {
                  n189 = local write "Recording"(FALSE ("Recording")) -> ()
                  n190 = Request Deallocation(TRUE ("标志")) -> ()
                }
                frame #1 {
                  n191 = Flush Queue(queue=w424) -> ()  [unwired: 1 in, 3 out]
                }
              }
            }
            frame "Blank stim" {
              n192 = flat-sequence {
                frame #0 {
                  n193 = Format Date/Time String() -> (date/time string=w505:string)  [unwired: 3 in]
                  n194 = local read "log"() -> (w500:string)
                  n195 = Concatenate Strings(w505, "\t", "show blank stim" ("字符串"), "\r", w500) -> (w502:string)
                  n196 = String Subset(string=w502, length (rest)=1000 ("y")) -> (substring=w501:string)  [unwired: 1 in]
                  n197 = local write "log"(w501) -> ()
                }
              }
              n198 = Number To Boolean Array(number="Pra_blank stim") -> (Boolean array=w496:bool[])
              n199 = call "Write_para_port0.vi"("port0（8元素）"=w496) -> ()  [unwired: 10 in, 1 out]
              n200 = local read "开始/暂停"() -> (w495:bool)
            }
            frame "ISI" {
              n201 = flat-sequence {
                tunnel: "Pra_ISI（ms）" -> [w512]
                tunnel: "Pra_ISI（ms）" -> [w519]
                frame #0 {
                  n202 = Number To Decimal String(number=w512) -> (decimal integer string=w516:string)  [unwired: 1 in]
                  n203 = Format Date/Time String() -> (date/time string=w518:string)  [unwired: 3 in]
                  n204 = local read "log"() -> (w511:string)
                  n205 = Concatenate Strings(w518, "\t", "ISI(ms)=" ("字符串"), w516, "\r", w511) -> (w514:string)
                  n206 = String Subset(string=w514, length (rest)=1000 ("y")) -> (substring=w513:string)  [unwired: 1 in]
                  n207 = local write "log"(w513) -> ()
                }
                frame #1 {
                  n208 = Wait (ms)(milliseconds to wait=w519) -> ()  [unwired: 1 out]
                }
              }
              n209 = local read "开始/暂停"() -> (w508:bool)
            }
            frame "wait", Default {
              n210 = Wait (ms)(milliseconds to wait="Pra_wait（ms）") -> ()  [unwired: 1 out]
              n211 = flat-sequence {
                tunnel: "Pra_wait（ms）" -> [w526]
                frame #0 {
                  n212 = Number To Decimal String(number=w526) -> (decimal integer string=w530:string)  [unwired: 1 in]
                  n213 = Format Date/Time String() -> (date/time string=w532:string)  [unwired: 3 in]
                  n214 = local read "log"() -> (w525:string)
                  n215 = Concatenate Strings(w532, "\t", "wait(ms)=" ("字符串"), w530, "\r", w525) -> (w528:string)
                  n216 = String Subset(string=w528, length (rest)=1000 ("y")) -> (substring=w527:string)  [unwired: 1 in]
                  n217 = local write "log"(w527) -> ()
                }
              }
              n218 = local read "开始/暂停"() -> (w522:bool)
            }
            frame "DR/R" {
              n219 = disable-structure shown="禁用" {
                frame Disabled {
                  n220 = flat-sequence {
                    frame #0 {
                      n221 = Format Date/Time String() -> (date/time string=w544:string)  [unwired: 3 in]
                      n222 = local read "log"() -> (w539:string)
                      n223 = Concatenate Strings(w544, "\t", "DR/R" ("字符串"), "\r", w539) -> (w541:string)
                      n224 = String Subset(string=w541, length (rest)=1000 ("y")) -> (substring=w540:string)  [unwired: 1 in]
                      n225 = local write "log"(w540) -> ()
                    }
                  }
                }
                frame Enabled {
                }
              }
              n226 = disable-structure shown="禁用" {
                disable-tunnel: w534 -> [w549 _]
                disable-tunnel: w533 -> [w548 _]
                frame Disabled {
                  n227 = local read item#-1() -> (w545)
                  n228 = Index Array(array=w545, index=w549) -> (element=w546)
                  n229 = call "dR.vi"() -> ("Image Dst Out"=w547:T1)  [unwired: 11 in]
                  n230 = case shown="0" w548 {
                    selector: w548 -> [_ w554]
                    tunnel: w547 -> [w551 w555]
                    tunnel: w546 -> [w550 w557]
                    frame 0 {
                      n231 = call "IMAQ Copy"("Image Dst"=w550, "Image Src"=w551) -> ()  [unwired: 4 in, 2 out]
                    }
                    frame 1, Default {
                      n232 = call "IMAQ Multiply"("Image Src A"=w557, "Constant"=w554, "Image Dst"=w557) -> ("Image Dst Out"=w556:T1)  [unwired: 4 in, 1 out]
                      n233 = Increment(x=w554) -> (x+1=w553:i32)
                      n234 = call "IMAQ Add"("Image Src A"=w556, "Image Dst"=w556, "Image Src B"=w555) -> ("Image Dst Out"=w552:T1)  [unwired: 4 in, 1 out]
                      n235 = call "IMAQ Divide"("Image Src A"=w552, "Constant"=w553, "Image Dst"=w552) -> ()  [unwired: 4 in, 2 out]
                    }
                  }
                }
                frame Enabled {
                }
              }
              n236 = local read "开始/暂停"() -> (w535:bool)
            }
            frame "wait heart" {
              n237 = flat-sequence {
                frame #0 {
                  n238 = Format Date/Time String() -> (date/time string=w567:string)  [unwired: 3 in]
                  n239 = local read "log"() -> (w562:string)
                  n240 = Concatenate Strings(w567, "\t", "wait heart" ("字符串"), "\r", w562) -> (w564:string)
                  n241 = String Subset(string=w564, length (rest)=1000 ("y")) -> (substring=w563:string)  [unwired: 1 in]
                  n242 = local write "log"(w563) -> ()
                }
              }
              n243 = local read "开始/暂停"() -> (w559:bool)
            }
            frame "wait calibrate" {
              n244 = local read "开始/暂停"() -> (w569:bool)
            }
            frame "openLightShutter" {
              n245 = flat-sequence {
                frame #0 {
                  n246 = Format Date/Time String() -> (date/time string=w579:string)  [unwired: 3 in]
                  n247 = local read "log"() -> (w574:string)
                  n248 = Concatenate Strings(w579, "\t", "open light shutter" ("字符串"), "\r", w574) -> (w576:string)
                  n249 = String Subset(string=w576, length (rest)=1000 ("y")) -> (substring=w575:string)  [unwired: 1 in]
                  n250 = local write "log"(w575) -> ()
                }
              }
              n251 = flat-sequence {
                frame #0 {
                  n252 = call "Write_para_port2_singalChange.vi"("索引"=1, "布尔"=TRUE) -> ()  [unwired: 9 in, 1 out]
                }
              }
              n253 = local read "开始/暂停"() -> (w571:bool)
            }
            frame "closeLightShutter" {
              n254 = flat-sequence {
                frame #0 {
                  n255 = Format Date/Time String() -> (date/time string=w591:string)  [unwired: 3 in]
                  n256 = local read "log"() -> (w586:string)
                  n257 = Concatenate Strings(w591, "\t", "close light shutter" ("字符串"), "\r", w586) -> (w588:string)
                  n258 = String Subset(string=w588, length (rest)=1000 ("y")) -> (substring=w587:string)  [unwired: 1 in]
                  n259 = local write "log"(w587) -> ()
                }
              }
              n260 = flat-sequence {
                frame #0 {
                  n261 = call "Write_para_port2_singalChange.vi"("索引"=1, "布尔"=FALSE) -> ()  [unwired: 9 in, 1 out]
                }
              }
              n262 = local read "开始/暂停"() -> (w583:bool)
            }
          }
        }
        "Stim_ID" <- w351
      }
      n263 = Flush File(refnum=w259) -> (refnum out=w258:refnum<file>)  [unwired: 1 in, 1 out]
      n264 = flat-sequence {
        tunnel: "Pra_DR/R parameter" -> [w288]
        tunnel: w258 -> [w287]
        tunnel: w263 -> [w286]
        frame #0 {
          n265 = local read "Pra_stim ID"() -> (w285:u8[])
          n266 = local read "FrameHeight"() -> (w273:i64)
          n267 = local read "FrameWidth"() -> (w274:i64)
          n268 = call "dR_R_ForFile.vi"("DR/R parameter"=w288, "stim ID"=w285, "OnlineMap"="Pra_OnlineMap", "blkIndex"=w286, "BlkFile"=w287) -> ("onLineMapOutput"=w283:T1[])  [unwired: 6 in]
          n269 = for {
            tunnel: w283 -> [w299] mode=indexing
            tunnel: w274 -> [w294]
            tunnel: w273 -> [_]
            i -> [w295]
            w297 = "write file data" ("替换字符串(\"\")")
            w303 = T4 0 items=["Grayscale (U8)", "Grayscale (I16)", "Grayscale (SGL)", "Complex (CSG)", "RGB (U32)", "HSL (U32)", "RGB (U64)", "Grayscale (U16)"] ("Image Type")
            n270 = Multiply(x=w295, y=w294) -> (x*y=w291:i64)
            n271 = Divide(x=w291, y=i64 2) -> (x/y=w289:dbl)
            n272 = Bundle(w289, "FrameHeight"=i64 0) -> (w293:cluster{dbl, "FrameHeight":i64})  [unwired: 1 in]
            n273 = call "IMAQ WindMove"("Window Number (0...15)"=w295, "Coordinates (screen)"=w293) -> ()  [unwired: 3 in, 2 out]
            n274 = call "IMAQ WindZoom 2"("Window Number (0...15)"=w295, "Zoom Factor"=sgl 0.5) -> ("error out"=w301:errorcluster)  [unwired: 6 in, 3 out]
            n275 = Number To Decimal String(number=w295, width (-)=i16 2 ("宽度(-)")) -> (decimal integer string=w312:string)
            n276 = call "IMAQ WindDraw"("Window Number (0...15)"=w295, "error in (no error)"=w301, "Title"=w299, "Image"=w299) -> ()  [unwired: 6 in, 2 out]
            n277 = local read "Pra_文件名"() -> (w314:string)
            n278 = call <vilib>:"Space Constant.vi"() -> ("String"=w311:string)
            n279 = call "IMAQ GetImageInfo"("Image"=w297) -> ("error out"=w298:errorcluster)  [unwired: 3 in, 7 out]
            n280 = Search and Replace String(replace all?=TRUE ("替换全部？(F)"), input string=w312, search string=w311, replace string="0" ("替换字符串(\"\")")) -> (result string=w307:string)  [unwired: 4 in, 3 out]
            n281 = case shown="错误" w298 {
              tunnel: w297 -> [w316 w318]
              tunnel: [w316 w317] -> w296
              frame No Error {
              }
              frame Error {
                w319 = T4 0 items=["Grayscale (U8)", "Grayscale (I16)", "Grayscale (SGL)", "Complex (CSG)", "RGB (U32)", "HSL (U32)", "RGB (U64)", "Grayscale (U16)"] ("Image Type")
                n282 = call "IMAQ Create"("Image Name"=w318, "Image Type"=w319) -> ("New Image"=w317:T1)  [unwired: 3 in, 1 out]
              }
            }
            n283 = local read "Pra_Blk目录"() -> (w300:path)
            n284 = Concatenate Strings(w314, "_" ("字符串"), w307, ".bmp" ("字符串")) -> (w305:string)
            n285 = call "IMAQ Cast Image"("Image Type"=w303, "Image Dst"=w296, "Image Src"=w299) -> ("Image Dst Out"=w302:T1)  [unwired: 7 in, 1 out]
            n286 = Build Path(base path=w300, name or relative path=w305) -> (appended path=w304:path)
            n287 = call-poly "IMAQ Write File 2"("File Path"=w304, "Image"=w302) -> ()  [unwired: 8 in, 2 out]
          }
          n288 = Format Date/Time String() -> (date/time string=w282:string)  [unwired: 3 in]
          n289 = local read "log"() -> (w277:string)
          n290 = Concatenate Strings(w282, "\t", "On Line Map" ("字符串"), "\r", w277) -> (w279:string)
          n291 = String Subset(string=w279, length (rest)=1000 ("y")) -> (substring=w278:string)  [unwired: 1 in]
          n292 = local write "log"(w278) -> ()
        }
      }
      "block" <- w263
    }
    n293 = local read "停止循环"() -> (w249:bool)
  }
  n294 = node-c288(w56) -> ()  [unwired: 1 out]
  n295 = call <vilib>:"Stop.vi"("error in (no error)"=w47, "Image In"=w52, "RefBrdIn"=w34) -> ("error out"=w48:errorcluster, "Image"=w51:T1, "RefBrdOut"=w33:u32)  [unwired: 6 in]
  n296 = call <vilib>:"Cleanup.vi"("error in (no error)"=w48, "Image In"=w51, "RefBrdIn"=w33) -> ("error out"=w49:errorcluster, "Image"=w50:T1, "RefBrdOut"=w32:u32)  [unwired: 6 in]
  n297 = call <vilib>:"Close.vi"("error in (no error)"=w49, "RefBrdIn"=w32) -> ("error out"=w31:errorcluster)  [unwired: 8 in, 1 out]
  n298 = call "Imaq Dispose"("Image"=w50, "error in (no error)"=w31) -> ("error out"=w12:errorcluster)  [unwired: 4 in]
  n299 = flat-sequence {
    tunnel: w12 -> [_]
    frame #0 {
      n300 = Stop(stop? (T)=TRUE ("停止？(T)")) -> ()
    }
  }
